vi "Align Impulses.vi"(0 "Data Input":T2 {"Data Channels" format="%.2f"}, 1 "Impulse Direction +ve?":bool, 2 "Alignment":enum16{"Vertically", "Horizontally"}(ring)=enum."Horizontally", 3 "Display":string, 4 "Impulse Plane":T3(ring), 5 "Impulse Positions (in)":T1(array[cluster]) {"Amplitude offset" format="%.2f"}, 9 "X Level":dbl format="%.2f", 11 "Y Level":dbl format="%.2f") -> (19 "Impulse Positions (out)":T1(array[cluster]) {"Amplitude offset" format="%.2f"})   [LabVIEW 2016, in "impulse functions.lvlib"]
uses:
  impulse functions.lvlib
panel:
  # "Copyright Americo A. Migliaccio (c) 2002 All Rights Reserved by Author"
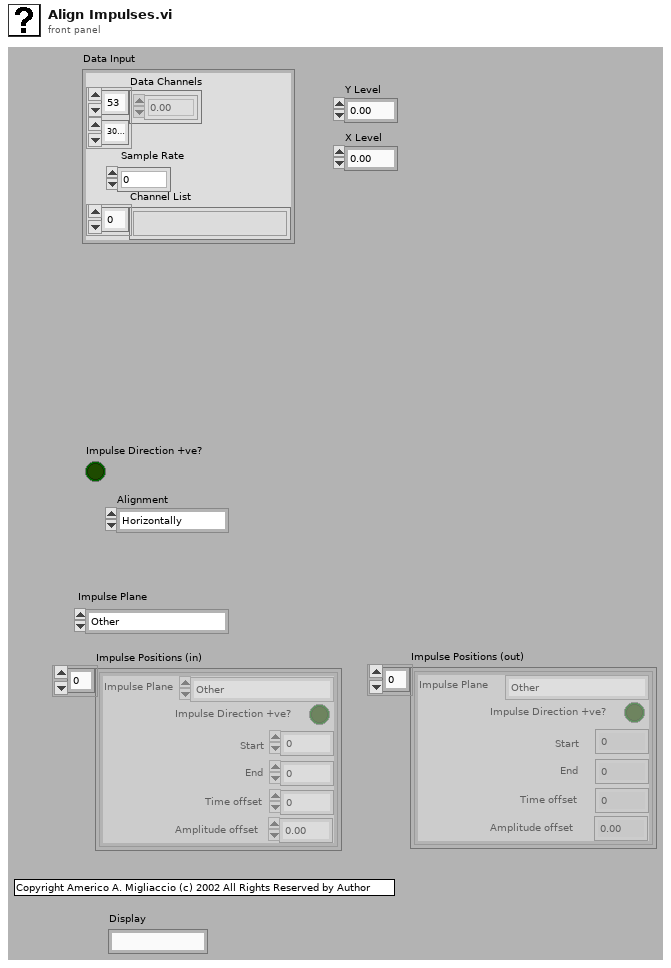
[diagram p1: front panel]
types:
  T1 = cluster{"Start":i32, "End":i32, "Impulse Plane":enum16{"Other", "Yaw", "Pitch", "Roll", "LARP", "RALP"}, "Impulse Direction +ve?":bool, "Time offset":i32, "Amplitude offset":dbl}[]
  T2 = cluster{"Data Channels":dbl[][], "Sample Rate":i32, "Channel List":string[]}
  T3 = enum16{"Other", "Yaw", "Pitch", "Roll", "LARP", "RALP"}
  T4 = cluster{"Start":i32, "End":i32, "Impulse Plane":enum16{"Yaw", "Pitch", "Roll", "LARP", "RALP"}, "Impulse Direction +ve?":bool, "Time offset":i32, "Amplitude offset":i32}[]
  T5 = cluster{"Start":i32, "End":i32, "Impulse Plane":u16, "Impulse Direction +ve?":bool, "Time offset":i32, "Amplitude offset":dbl}[]
  T6 = cluster{"Start":i32, "End":i32, "Impulse Plane":enum16{"Other", "Yaw", "Pitch", "Roll", "LARP", "RALP"}, "Impulse Direction +ve?":bool, "Time offset":i32, "Amplitude offset":dbl}
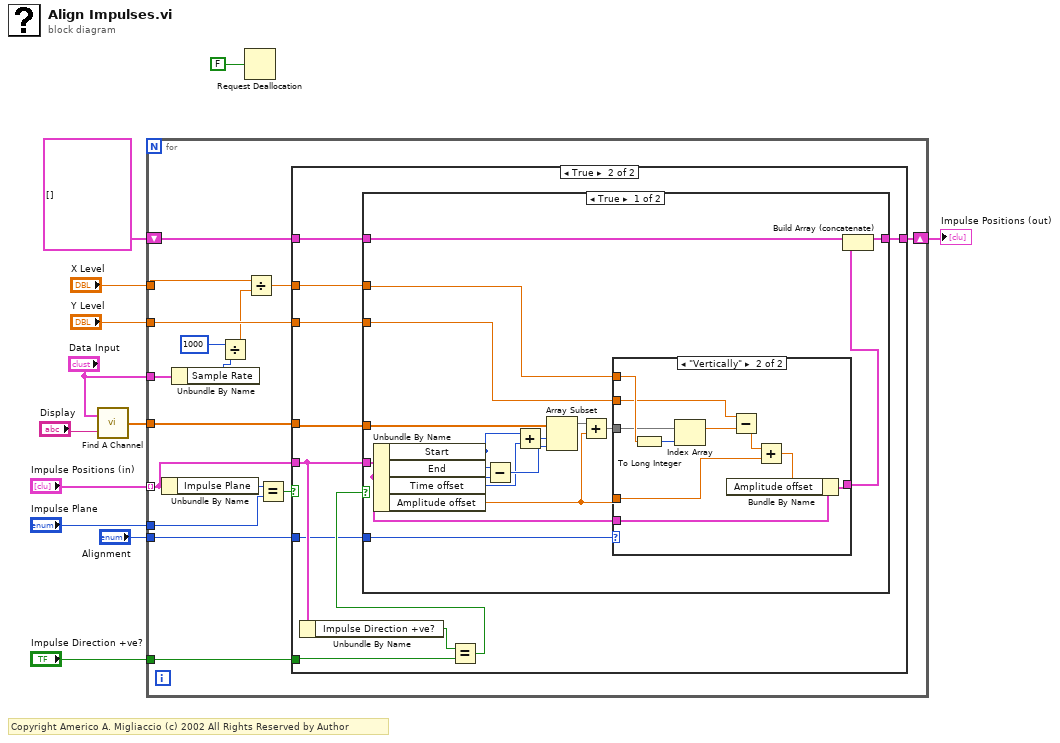
[diagram p0: block diagram]
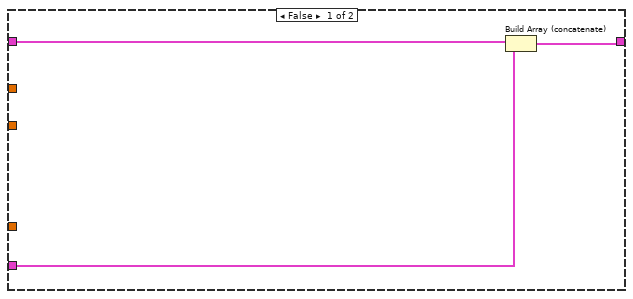
[diagram p2: hidden frame]
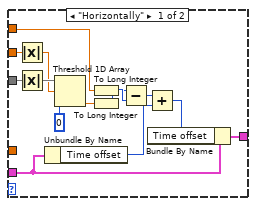
[diagram p3: hidden frame]
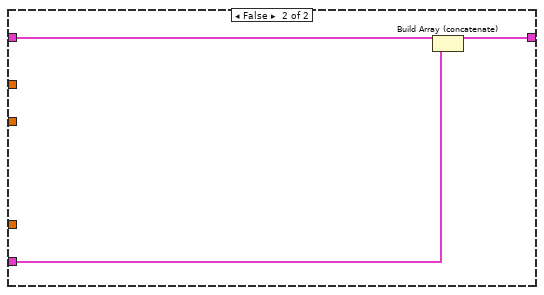
[diagram p4: hidden frame]
diagram:
  # "Copyright Americo A. Migliaccio (c) 2002 All Rights Reserved by Author"
  n1 = call "Find A Channel.vi"("element"="Display", "Data Output"="Data Input") -> ("Signal (V)"=w9:dbl[])
  n2 = for {
    tunnel: "Impulse Positions (in)" -> [w25] mode=indexing
    tunnel: "Impulse Plane" -> [w27]
    tunnel: w9 -> [w24]
    tunnel: "Impulse Direction +ve?" -> [w23]
    shift-right: [w20] -> w5
    shift-left: T4 [] -> [w21]
    tunnel: "Y Level" -> [w22]
    tunnel: "X Level" -> [w14]
    tunnel: "Alignment" -> [w19]
    tunnel: "Data Input" -> [w18]
    n3 = Unbundle By Name(w25) -> ("Impulse Plane"=w28:T3)
    n4 = Unbundle By Name(w18) -> ("Sample Rate"=w16:i32)
    n5 = Divide(x=1000, y=w16) -> (x/y=w13:dbl)
    n6 = Divide(x=w14, y=w13) -> (x/y=w17:dbl)
    n7 = Equal?(x=w28, y=w27) -> (x = y?=w26:bool)
    n8 = case shown="True" w26 {
      tunnel: w25 -> [w29 w40]
      tunnel: w24 -> [_ w41]
      tunnel: w23 -> [_ w39]
      tunnel: w22 -> [_ w36]
      tunnel: w17 -> [_ w35]
      tunnel: w21 -> [w31 w34]
      tunnel: [w30 w33] -> w20
      tunnel: w19 -> [_ w32]
      frame False {
        n9 = Build Array (concatenate)(w31, w29) -> (w30:T5)
      }
      frame True {
        n10 = Unbundle By Name(w40) -> ("Impulse Direction +ve?"=w37:bool)
        n11 = Equal?(x=w37, y=w39) -> (x = y?=w38:bool)
        n12 = case shown="True" w38 {
          tunnel: w40 -> [w55 w82]
          tunnel: w41 -> [w56 _]
          tunnel: w36 -> [w47 _]
          tunnel: w35 -> [w48 _]
          tunnel: w34 -> [w52 w84]
          tunnel: [w51 w83] -> w33
          tunnel: w32 -> [w49 _]
          frame True {
            n13 = Unbundle By Name(w55) -> ("Start"=w45:i32, "End"=w54:i32, "Time offset"=w44:i32, "Amplitude offset"=w42:dbl)
            n14 = Subtract(x=w54, y=w45) -> (x-y=w57:i32)
            n15 = Add(x=w45, y=w44) -> (x+y=w46:i32)
            n16 = Array Subset(array=w56, index=w46, length=w57) -> (w50:dbl[])
            n17 = Add(x=w50, y=w42) -> (x+y=w43:dbl[])
            n18 = case shown="\"Vertically\"" w49 {
              tunnel: w55 -> [w62 w77]
              tunnel: w48 -> [w65 w80]
              tunnel: [w63 w76] -> w53
              tunnel: w43 -> [w67 w79]
              tunnel: w47 -> [w70 w78]
              tunnel: w42 -> [_ w73]
              frame "Horizontally" {
                n19 = Absolute Value(x=w70) -> (abs(x)=w68:dbl)
                n20 = Absolute Value(x=w67) -> (abs(x)=w71:dbl[])
                n21 = Unbundle By Name(w62) -> ("Time offset"=w60:i32)
                n22 = Threshold 1D Array(1:0 ("start index (0)"), 2:w68, 3:w71) -> (0:w64:dbl)
                n23 = To Long Integer(number=w65) -> (32bit integer=w59:i32)
                n24 = To Long Integer(number=w64) -> (32bit integer=w58:i32)
                n25 = Subtract(x=w58, y=w59) -> (x-y=w66:i32)
                n26 = Add(x=w66, y=w60) -> (x+y=w61:i32)
                n27 = Bundle By Name(cluster=w62, "Time offset"=w61) -> (w63:T6)
              }
              frame "Vertically" {
                n28 = To Long Integer(number=w80) -> (32bit integer=w81:i32)
                n29 = Index Array(array=w79, index=w81) -> (element=w75:dbl)
                n30 = Subtract(x=w78, y=w75) -> (x-y=w74:dbl)
                n31 = Add(x=w74, y=w73) -> (x+y=w72:dbl)
                n32 = Bundle By Name(cluster=w77, "Amplitude offset"=w72) -> (w76:T6)
              }
            }
            n33 = Build Array (concatenate)(w52, w53) -> (w51:T5)
          }
          frame False {
            n34 = Build Array (concatenate)(w84, w82) -> (w83:T5)
          }
        }
      }
    }
  }
  "Impulse Positions (out)" <- w5
  n35 = Request Deallocation(FALSE ("flag")) -> ()
